vi "GetBoardCenter.vi"(8 "error in (no error)":errorcluster, 11 "Board in":refnum<class "Board.lvclass">) -> (0 "error out":errorcluster, 2 "Center":T1, 3 "Board out":refnum<class "Board.lvclass">)   [LabVIEW 2015, in "TronviewGame.lvlib" / "Board.lvclass"]
uses:
  Board.lvclass
  Position.ctl
  Board.lvclass/Board.ctl
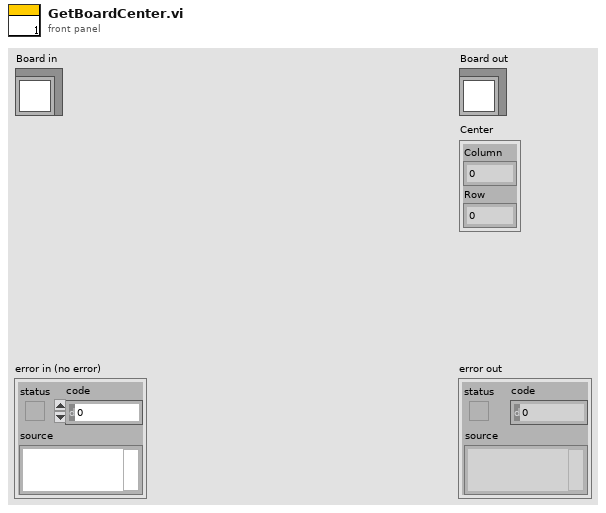
[diagram p1: front panel]
types:
  T1 = typedef "TronviewGame.lvlib/Board.lvclass/Position.ctl" = cluster{"Column":i32, "Row":i32}
  T2 = typedef "TronviewGame.lvlib/Board.lvclass/BoardSize.ctl" = cluster{"Columns":u32, "Rows":u32}
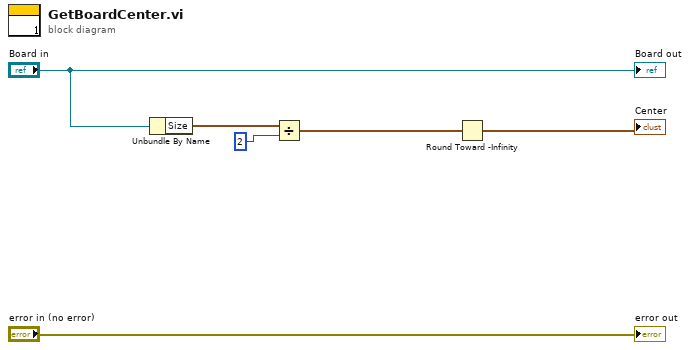
[diagram p0: block diagram]
diagram:
  n1 = Unbundle By Name("Board in") -> ("Size"=w1:T2)
  n2 = Divide(x=w1, y=2) -> (x/y=w3:cluster{"Columns":dbl, "Rows":dbl})
  n3 = Round Toward -Infinity(1:w3) -> (0:→"Center":cluster{"Columns":dbl, "Rows":dbl})
  "error out" <- "error in (no error)"
  "Board out" <- "Board in"
